vi "Update Sync delay value_2021.vi"() -> (0 "error out":errorcluster, 4 "Path":path)   [LabVIEW 2020]
panel:
  out "Array":path[](array[path])
  out "File Changed":bool
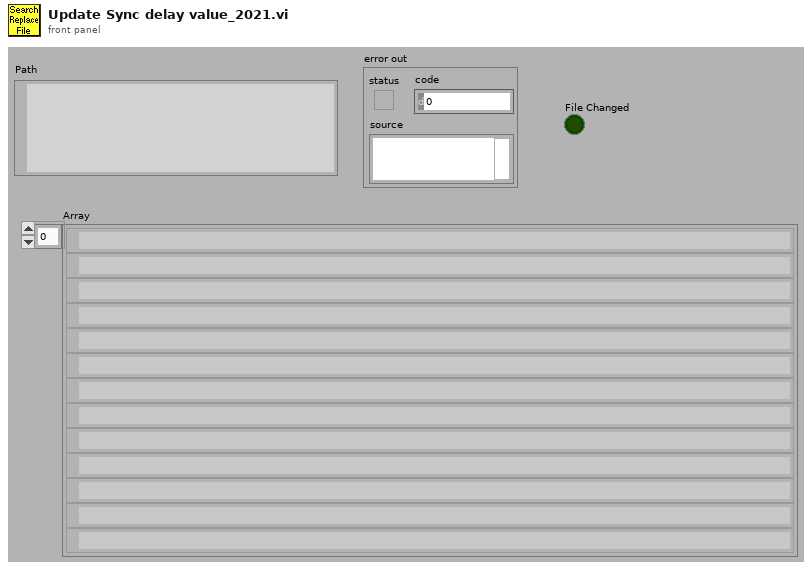
[diagram p1: front panel]
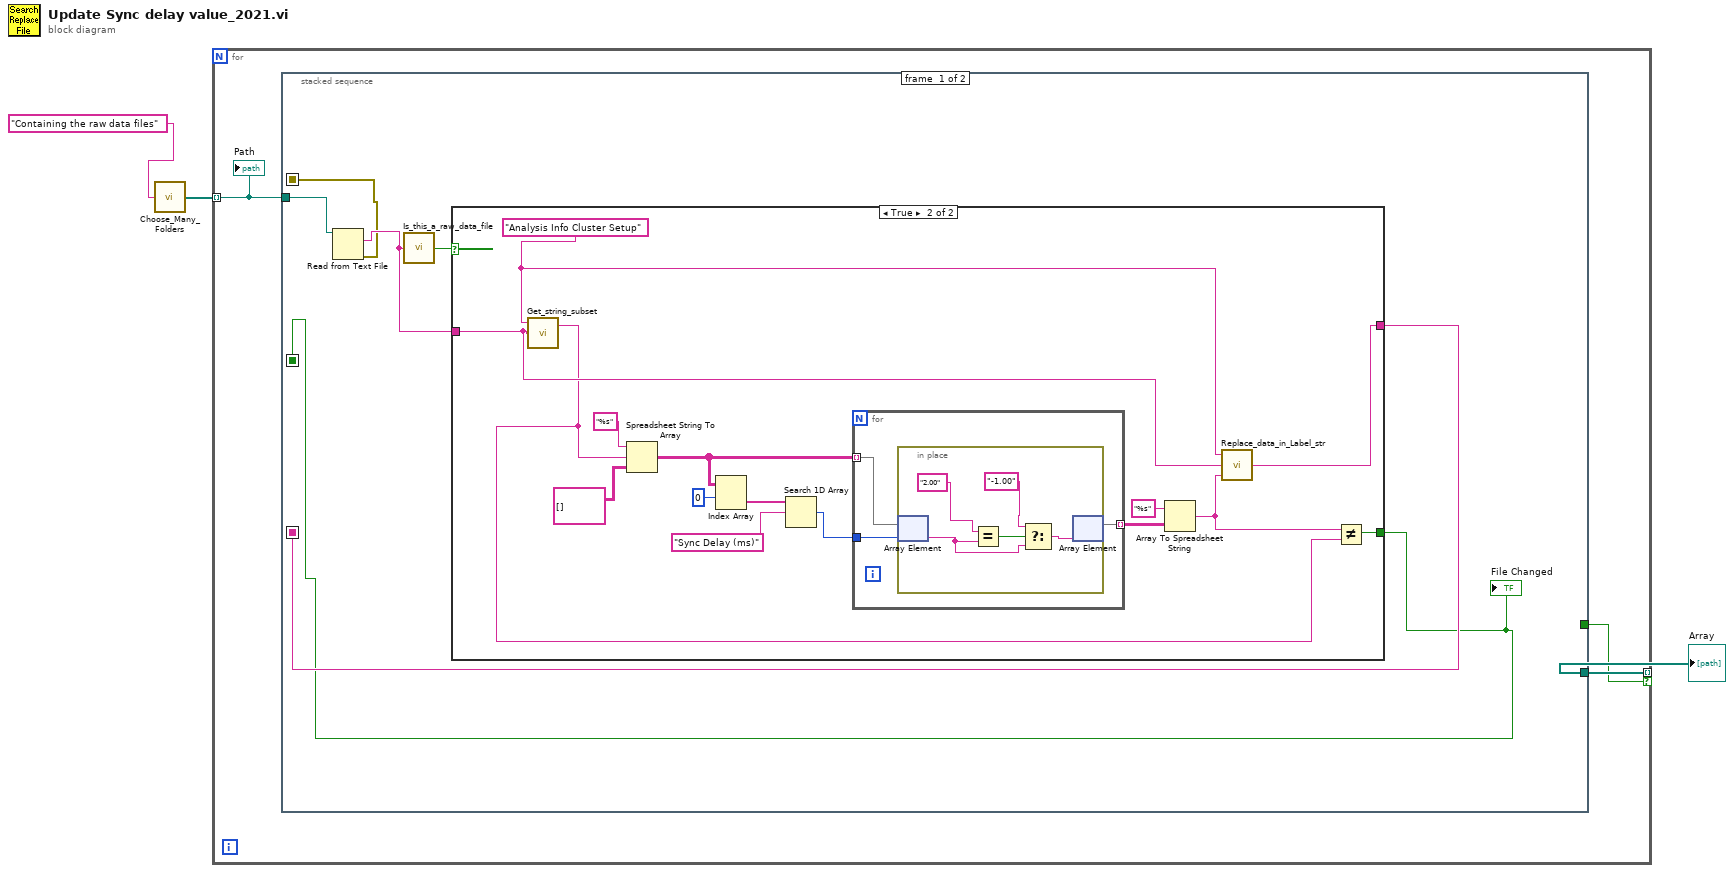
[diagram p0: block diagram]
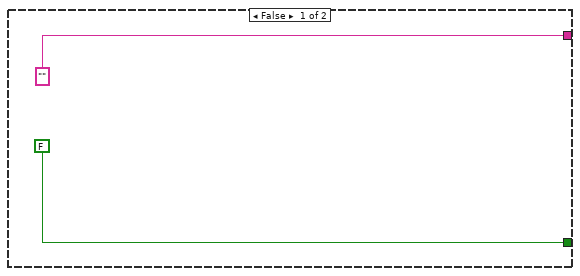
[diagram p2: hidden frame]
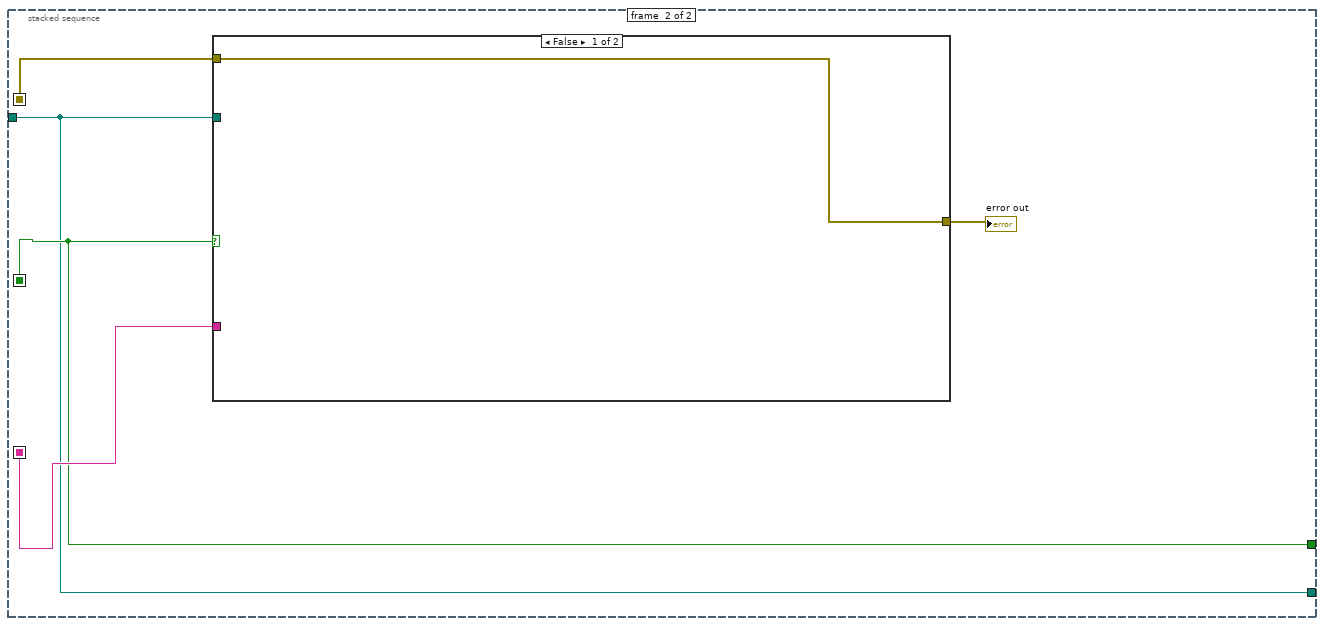
[diagram p3: hidden frame]
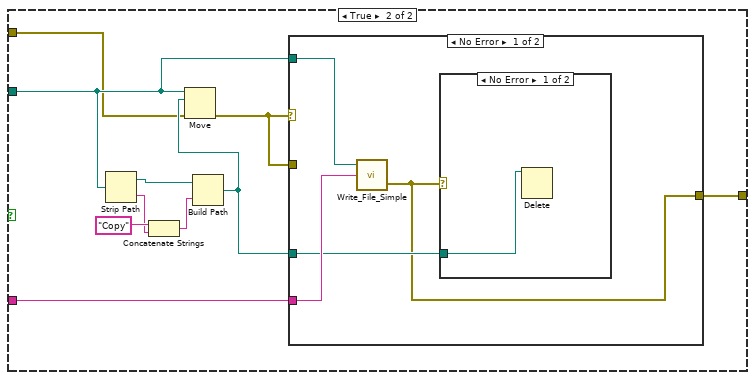
[diagram p4: hidden frame]
diagram:
  n1 = call "Choose_Many_Folders.vi"("Purpose of choosing folder"="Containing the raw data files") -> ("Files"=w2:path[])
  n2 = for {
    tunnel: w2 -> [w6] mode=indexing
    tunnel: [w5] -> w1 mode=indexing if=w4
    n3 = stacked-sequence {
      seq-local: [w7 _] -> [_ w41]
      seq-local: [w12 _] -> [_ w40]
      seq-local: [w11 _] -> [_ w39]
      tunnel: w6 -> [w10 w38]
      tunnel: [_ w38] -> w5
      tunnel: [_ w39] -> w4
      frame #0 {
        n4 = Read from Text File(file (use dialog)=w10) -> (text=w8:string, error out=w7:errorcluster)  [unwired: 3 in, 2 out]
        n5 = call "Is_this_a_raw_data_file.vi"("character string"=w8) -> ("Raw Dat File?"=w9:bool)  [unwired: 2 out]
        n6 = case shown="True" w9 {
          tunnel: ["" ("string") w18] -> w12
          tunnel: [FALSE w15] -> w11
          tunnel: w8 -> [_ w20]
          frame False {
          }
          frame True {
            w19 = "Analysis Info Cluster Setup"
            n7 = call "Get_string_subset.vi"("String to split"=w20, "File Label"=w19) -> ("Output string"=w16:string)  [unwired: 2 in, 1 out]
            n8 = Spreadsheet String To Array(format string="%s", spreadsheet string=w16, array type (2D Dbl)=string[][] []) -> (array=w27:string[][])  [unwired: 1 in]
            n9 = Index Array(array=w27, index (row)=0) -> (element=w25:string[])  [unwired: 1 in]
            n10 = Search 1D Array(1D array=w25, element="Sync Delay (ms)") -> (index of element=w26:i32)  [unwired: 1 out]
            n11 = for {
              tunnel: w26 -> [w31]
              tunnel: w27 -> [w32] mode=indexing
              tunnel: [w30] -> w29 mode=indexing
              n12 = in-place {
                n13 = in-place-array #1 ("Array Index / Replace Elements")(w32, w31) -> (w34:string)
                n14 = Equal?(x="2.00", y=w34) -> (x = y?=w36:bool)
                n15 = Select(t="-1.00", s=w36, f=w34) -> (s? t:f=w33:string)
                n16 = in-place-array #1(w33) -> (w30:string[])  [unwired: 1 out]
              }
            }
            n17 = Array To Spreadsheet String(array=w29, 3:"%s" ("format string")) -> (spreadsheet string=w17:string)  [unwired: 1 in]
            n18 = call "Replace_data_in_Label_str.vi"("New data string"=w17, "Input string"=w20, "Variable name"=w19) -> ("Appended string"=w18:string)
            n19 = Not Equal?(x=w17, y=w16) -> (x != y?=w15:bool)
          }
        }
        "File Changed" <- w11
      }
      frame #1 {
        n20 = case shown="False" w39 {
          tunnel: w38 -> [_ w49]
          tunnel: w40 -> [_ w48]
          tunnel: [w43 w46] -> w42
          tunnel: w41 -> [w43 w44]
          frame False {
          }
          frame True {
            n21 = Strip Path(path=w49) -> (stripped path=w50:path, name=w52:string)
            n22 = Concatenate Strings("Copy" ("name or relative path"), w52) -> (w51:string)
            n23 = Build Path(base path=w50, name or relative path=w51) -> (appended path=w47:path)
            n24 = Move(source path=w49, error in=w44, 10:w47) -> (error out=w45:errorcluster)  [unwired: 2 in, 2 out]
            n25 = case shown="No Error" w45 {
              tunnel: w49 -> [w57 _]
              tunnel: w48 -> [w56 _]
              tunnel: w47 -> [w55 _]
              tunnel: [w54 w59] -> w46
              tunnel: w45 -> [_ w59]
              frame No Error {
                n26 = call "Write_File_Simple.vi"("character string"=w56, "file path"=w57) -> ("error out"=w54:errorcluster)  [unwired: 1 in, 1 out]
                n27 = case shown="No Error" w54 {
                  tunnel: w55 -> [w58 _]
                  frame No Error {
                    n28 = Delete(path (use dialog)=w58) -> ()  [unwired: 4 in, 3 out]
                  }
                  frame Error {
                  }
                }
              }
              frame Error {
              }
            }
          }
        }
        "error out" <- w42
      }
    }
    "Path" <- w6
  }
  "Array" <- w1
